vi "20[1]-S7F1 Function.vi"(8 "error in (no error)":errorcluster, 10 "SECS-II Class":refnum<class "SECS-II Class.lvclass">, 11 "20-Process Program Downloading in":refnum<class "20-Process Program Downloading.lvclass">) -> (0 "error out":errorcluster, 2 "SECS-II Class Out":refnum<class "SECS-II Class.lvclass">, 3 "20-Process Program Downloading out":refnum<class "20-Process Program Downloading.lvclass">)   [LabVIEW 2020, in "SECS Scenarios.lvlib" / "20-Process Program Downloading.lvclass"]
uses:
  20-Process Program Downloading.lvclass
  D:/Dropbox/SECS/SECS_GEM v1.1.0/Com/SECS Scenarios/Scenarios Class/Scenarios Class.lvclass
  SECS Communication/SECS-II Class/SECS-II Class.lvclass
  SECS Communication/S7 Message Class/S7 Message Class.lvclass
  D:/Dropbox/SECS/SECS_GEM v1.1.0/Com/SECS Communication/SECS-II Class/SECS-II Class.lvclass
  Scenarios Class/Reply State.ctl
  Scenarios Class/Scenarios Class.lvclass/Scenarios Class.ctl
  Scenarios Class/Write Reply State.vi
  Scenarios Class/Read HSMS Class.vi
  SECS Communication/HSMS Class/HSMS Class.lvclass
  Scenarios Class/Scenarios Class.lvclass
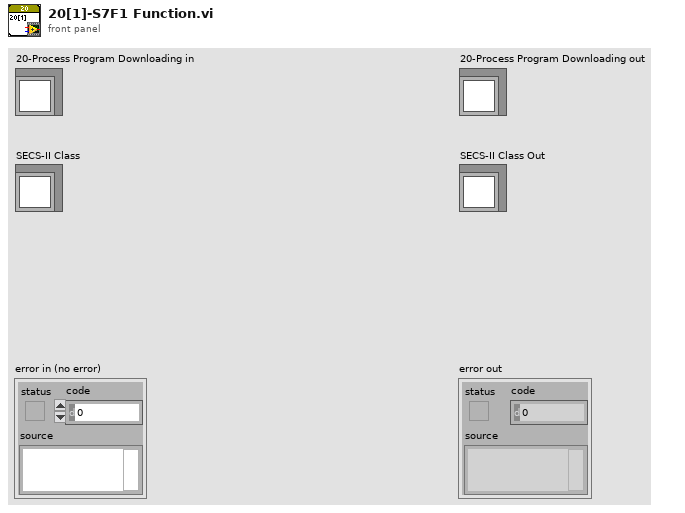
[diagram p1: front panel]
types:
  T1 = typedef "SECS Communication.lvlib/S7 Message Class.lvclass/S7F1.ctl" = cluster{"PPID":string, "LENGTH":u32}
  T2 = typedef "SECS Scenarios.lvlib/Scenarios Class.lvclass/Reply State.ctl" = enum16{"OK", "Illegal Data", "Unknown Stream", "Unknown Function", "Off-Line", "T3 Timeout", "Inner-Timeout"}
  T3 = typedef "SECS Communication.lvlib/S7 Message Class.lvclass/S7F2.ctl" = enum8{"Ok", "already have", "no space", "invalid PPID", "busy, try later", "will not accept", " other error"}
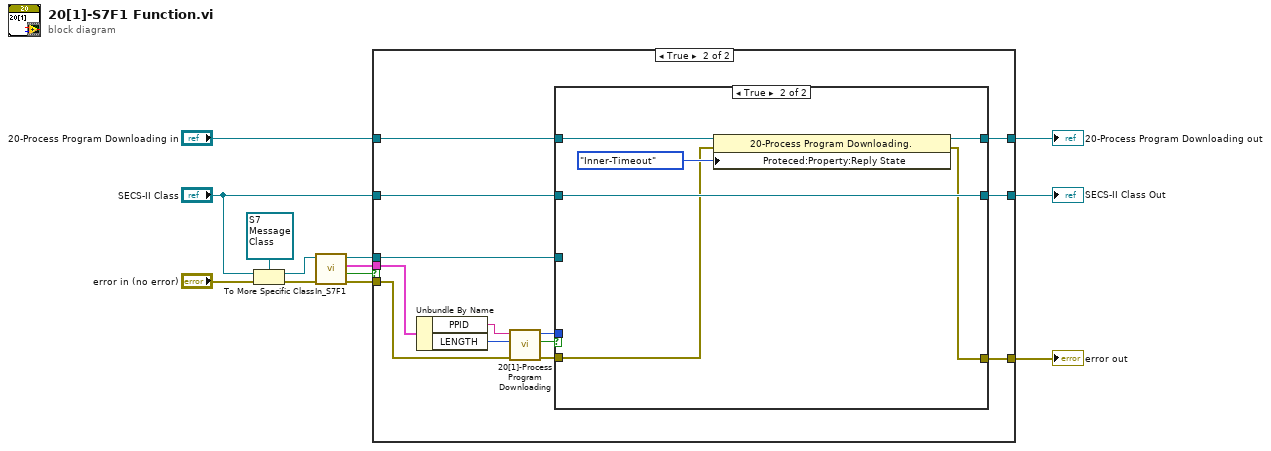
[diagram p0: block diagram]
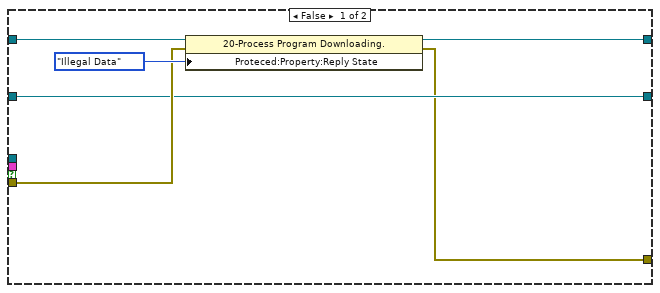
[diagram p2: hidden frame]
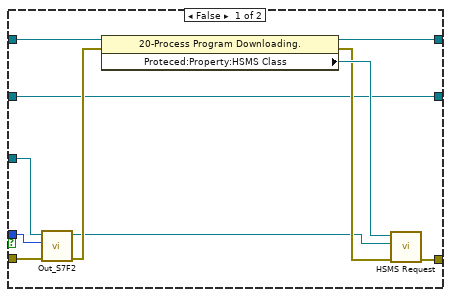
[diagram p3: hidden frame]
diagram:
  n1 = To More Specific Class(target class=refnum<class "S7 Message Class.lvclass"> refnum ("S7 Message Class in"), reference="SECS-II Class", error in="error in (no error)") -> (specific class reference=w11:refnum<class "S7 Message Class.lvclass">, error out=w12:errorcluster)
  n2 = call "In_S7F1.vi"("error in (no error)"=w12, "S7 Message Class in"=w11) -> ("error out"=w10:errorcluster, "OK?"=w1:bool, "S7F1"=w9:T1, "S7 Message Class out"=w8:refnum<class "S7 Message Class.lvclass">)  [unwired: 6 in]
  n3 = case shown="True" w1 {
    tunnel: w10 -> [w17 w32]
    tunnel: w9 -> [_ w31]
    tunnel: w8 -> [_ w28]
    tunnel: "20-Process Program Downloading in" -> [w19 w24]
    tunnel: [w14 w23] -> w5
    tunnel: [w16 w22] -> w4
    tunnel: "SECS-II Class" -> [w15 w21]
    tunnel: [w15 w20] -> w2
    frame False {
      n4 = property class="20-Process Program Downloading."(reference=w19, error in=w17, "Proteced:Property:Reply State"=Reply_State."Illegal Data" ("Reply State")) -> (reference out=w16:refnum<class "20-Process Program Downloading.lvclass">, error out=w14:errorcluster)
    }
    frame True {
      n5 = Unbundle By Name(w31) -> ("PPID"=w29:string, "LENGTH"=w30:u32)
      n6 = call "20[1]-Process Program Downloading.vi"("error in (no error)"=w32, "LENGTH"=w30, "PPID"=w29) -> ("error out"=w27:errorcluster, "Timeout?"=w25:bool, "S7F2"=w26:T3)  [unwired: 6 in]
      n7 = case shown="True" w25 {
        tunnel: w24 -> [w43 w47]
        tunnel: w28 -> [w37 _]
        tunnel: [w40 w44] -> w23
        tunnel: [w39 w45] -> w22
        tunnel: w27 -> [w38 w46]
        tunnel: w26 -> [w34 _]
        tunnel: w21 -> [w33 w49]
        tunnel: [w33 w49] -> w20
        frame False {
          n8 = call "Out_S7F2.vi"("error in (no error)"=w38, "S7F2"=w34, "S7 Message Class in"=w37) -> ("error out"=w36:errorcluster, "S7 Message Class out"=w35:refnum<class "S7 Message Class.lvclass">)  [unwired: 7 in]
          n9 = property class="20-Process Program Downloading."(reference=w43, error in=w36) -> (reference out=w39:refnum<class "20-Process Program Downloading.lvclass">, error out=w41:errorcluster, "Proteced:Property:HSMS Class"=w42:refnum<class "HSMS Class.lvclass">)
          n10 = call "HSMS Request.vi"("error in (no error)"=w41, "SECS-II Class In"=w35, "HSMS Class in"=w42) -> ("error out"=w40:errorcluster)  [unwired: 7 in, 1 out]
        }
        frame True {
          n11 = property class="20-Process Program Downloading."(reference=w47, error in=w46, "Proteced:Property:Reply State"=Reply_State."Inner-Timeout" ("Reply State")) -> (reference out=w45:refnum<class "20-Process Program Downloading.lvclass">, error out=w44:errorcluster)
        }
      }
    }
  }
  "error out" <- w5
  "20-Process Program Downloading out" <- w4
  "SECS-II Class Out" <- w2
